vi "calculate pulse statistics.vi"(8 "error in (no error)":errorcluster, 9 "gain":dbl=1.0, 10 "crossing stats":T1, 11 "display queues":T2) -> (0 "error out":errorcluster)   [LabVIEW 2017]
uses:
  typedefs/queue cluster.ctl
  typedefs/reading queue.ctl
  typedefs/reading.ctl
  typedefs/readingType.ctl
  typedefs/reading 1 queue.ctl
  typedefs/reading1.ctl
  popup panels/control panel globals.vi
  <vilib>/Analysis/NI_AALPro.lvlib
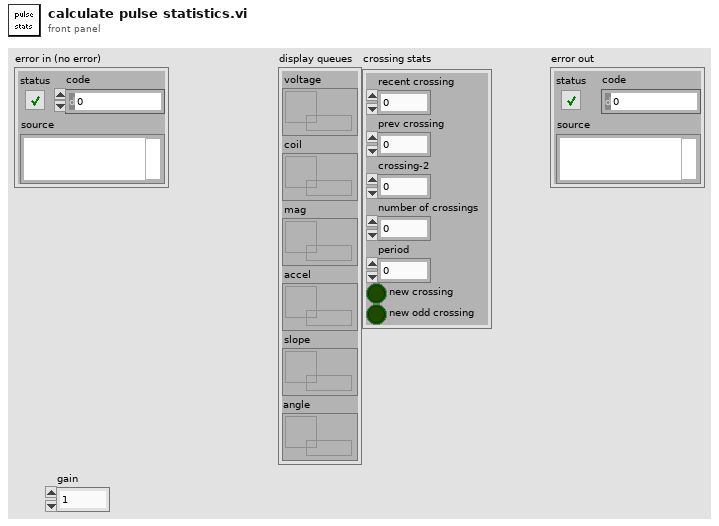
[diagram p1: front panel]
types:
  T1 = cluster{"recent crossing":dbl, "prev crossing":dbl, "crossing-2":dbl, "number of crossings":i32, "period":dbl, "new crossing":bool, "new odd crossing":bool}
  T2 = typedef "queue cluster.ctl" = cluster{"voltage":T3, "coil":T3, "mag":T3, "accel":T3, "slope":T4, "angle":T3}
  T3 = typedef "reading queue.ctl" = refnum<queue>
  T4 = typedef "reading 1 queue.ctl" = refnum<queue>
  T5 = typedef "reading.ctl" = cluster{"reading type":T6, "time":fxp<+,48,48>, "x":sgl, "y":sgl, "z":sgl, "XSUM":u8}
  T6 = typedef "readingType.ctl" = enum8{"SYNC", "DETVAL", "COILI", "MAGVEC", "ACCVEC"}
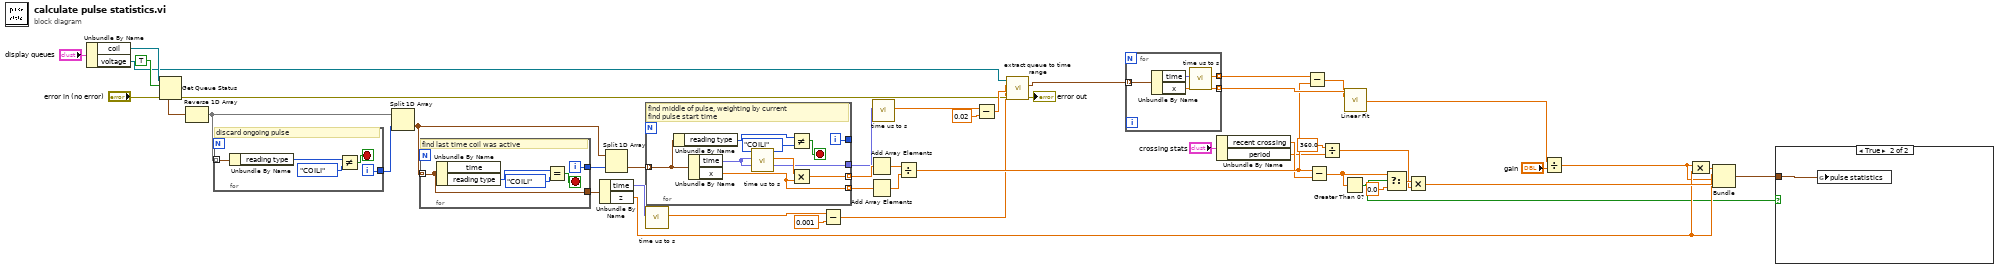
[diagram p0: block diagram]
diagram:
  n1 = Unbundle By Name("display queues") -> ("coil"=w31:T3, "voltage"=w26:T3)
  n2 = Get Queue Status(queue=w31, return elements? (F)=TRUE, error in (no error)="error in (no error)") -> (error out=w25:errorcluster, elements=w29:T5[])  [unwired: 6 out]
  n3 = Reverse 1D Array(array=w29) -> (reversed array=w45:T5[])
  n4 = for {
    tunnel: w45 -> [w49] mode=indexing
    tunnel: [w48] -> w44
    i -> [w48]
    stop <- w50 stop-if-true
    # "discard ongoing pulse"
    n5 = Unbundle By Name(w49) -> ("reading type"=w52:T6)
    n6 = Not Equal?(x=w52, y=readingType."COILI") -> (x != y?=w50:bool)
  }
  n7 = Split 1D Array(array=w45, index=w44) -> (second subarray=w43:T5[])  [unwired: 1 out]
  n8 = for {
    tunnel: w43 -> [w54] mode=indexing
    tunnel: [w54] -> w47
    tunnel: [w53] -> w42
    i -> [w53]
    stop <- w55 stop-if-true
    # "find last time coil was active"
    n9 = Unbundle By Name(w54) -> ("reading type"=w57:T6)  [unwired: 1 out]
    n10 = Equal?(x=w57, y=readingType."COILI") -> (x = y?=w55:bool)
  }
  n11 = Unbundle By Name(w47) -> ("time"=w15:fxp<+,48,48>, "z"=w10:sgl)
  n12 = Split 1D Array(array=w43, index=w42) -> (second subarray=w41:T5[])  [unwired: 1 out]
  n13 = for {
    tunnel: w41 -> [w63] mode=indexing
    tunnel: [w62] -> w21 mode=indexing
    tunnel: [w61] -> w20 mode=indexing
    tunnel: [w59] -> w16
    tunnel: [w58] -> _
    i -> [w58]
    stop <- w64 stop-if-true
    # "find middle of pulse, weighting by current\nfind pulse start time"
    n14 = Unbundle By Name(w63) -> ("reading type"=w66:T6)
    n15 = Unbundle By Name(w63) -> ("time"=w59:fxp<+,48,48>, "x"=w61:sgl)
    n16 = call "time us to s.vi"("time (us)"=w59) -> ("time (s)"=w60:dbl)  [unwired: 10 in]
    n17 = Not Equal?(x=w66, y=readingType."COILI") -> (x != y?=w64:bool)
    n18 = Multiply(x=w60, y=w61) -> (x*y=w62:dbl)
  }
  n19 = call "time us to s.vi"("time (us)"=w15) -> ("time (s)"=w14:dbl)  [unwired: 10 in]
  n20 = Subtract(x=w14, y=0.001) -> (x-y=w12:dbl)
  n21 = Add Array Elements(numeric array=w21) -> (sum=w19:dbl)
  n22 = Add Array Elements(numeric array=w20) -> (sum=w18:sgl)
  n23 = call "time us to s.vi"("time (us)"=w16) -> ("time (s)"=w13:dbl)  [unwired: 10 in]
  n24 = Divide(x=w19, y=w18) -> (x/y=w17:dbl)
  n25 = Subtract(x=w13, y=0.02) -> (x-y=w27:dbl)
  n26 = call "extract queue to time range.vi"("error in (no error)"=w25, "t0"=w27, "t1"=w12, "queue"=w26) -> ("error out"=→"error out":errorcluster, "extracted data"=w22:T5[])  [unwired: 6 in]
  n27 = for {
    tunnel: w22 -> [w69] mode=indexing
    tunnel: [w67] -> w40 mode=indexing
    tunnel: [w70] -> w39 mode=indexing
    n28 = Unbundle By Name(w69) -> ("time"=w68:fxp<+,48,48>, "x"=w70:sgl)
    n29 = call "time us to s.vi"("time (us)"=w68) -> ("time (s)"=w67:dbl)  [unwired: 10 in]
  }
  n30 = Unbundle By Name("crossing stats") -> ("recent crossing"=w8:dbl, "period"=w7:dbl)
  n31 = Subtract(x=w40, y=w17) -> (x-y=w38:dbl[])
  n32 = Subtract(x=w17, y=w8) -> (x-y=w5:dbl)
  n33 = Divide(x=360.0, y=w7) -> (x/y=w34:dbl)
  n34 = Greater Than 0?(x=w5) -> (x > 0?=w1:bool)
  n35 = call <vilib>:"Linear Fit.vi"("Y"=w39, "X"=w38) -> ("intercept"=w4:dbl)  [unwired: 9 in, 4 out]
  n36 = Select(t=w5, s=w1, f=0.0) -> (s? t:f=w36:dbl)
  n37 = Multiply(x=w36, y=w34) -> (x*y=w33:dbl)
  n38 = Divide(x=w4, y="gain") -> (x/y=w3:dbl)
  n39 = Compound Arithmetic op=MULTIPLY(w3, w10) -> (w2:dbl)
  n40 = Bundle(w2, w33, w3, "z"=w10) -> (w6:cluster{dbl, dbl, dbl, "z":sgl})  [unwired: 1 in]
  n41 = case shown="True" w1 {
    tunnel: w6 -> [_ w71]
    frame False {
    }
    frame True {
      n42 = global write "control panel globals.vi" "pulse statistics"(w71) -> ()
    }
  }
